vi "ListExamples.vi"(10 "Folder":string) -> (0 "VI Paths":path[](array[path]), 1 "Paths":path[](array[path]), 2 "vis":string[](array[string]), 3 "filenames":string[](array[string]), 5 "folder names":string[](array[string]))   [LabVIEW 2020]
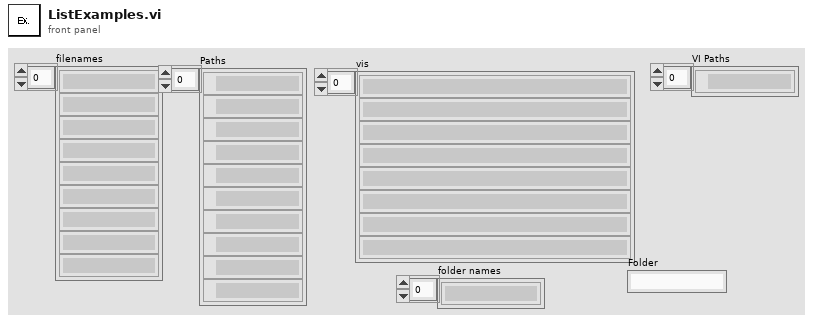
[diagram p1: front panel]
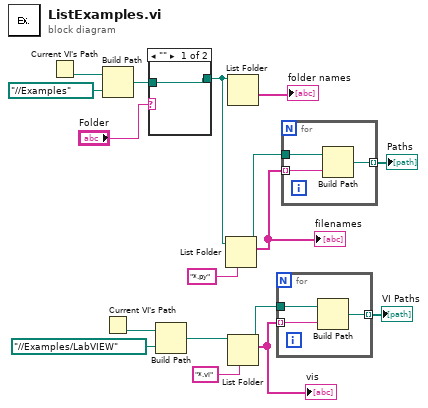
[diagram p0: block diagram]
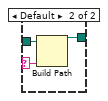
[diagram p2: hidden frame]
diagram:
  n1 = Current VI's Path() -> (path=w5:path)
  n2 = Build Path(base path=w5, name or relative path=path "../../Examples") -> (appended path=w3:path)
  n3 = Current VI's Path() -> (path=w12:path)
  n4 = case shown="\"\"" "Folder" {
    selector: "Folder" -> [_ w19]
    tunnel: w3 -> [w18 w21]
    tunnel: [w18 w20] -> w2
    frame "" {
    }
    frame Default {
      n5 = Build Path(base path=w21, name or relative path=w19) -> (appended path=w20:path)
    }
  }
  n6 = Build Path(base path=w12, name or relative path=path "../../Examples/LabVIEW") -> (appended path=w11:path)
  n7 = List Folder(path=w2, pattern="*.py") -> (path out=w16:path, filenames=w15:string[])  [unwired: 2 in, 2 out]
  "filenames" <- w15
  n8 = List Folder(path=w2) -> (folder names=→"folder names":string[])  [unwired: 3 in, 3 out]
  n9 = List Folder(path=w11, pattern="*.vi") -> (path out=w10:path, filenames=w9:string[])  [unwired: 2 in, 2 out]
  "vis" <- w9
  n10 = for {
    tunnel: w10 -> [w24]
    tunnel: w9 -> [w23] mode=indexing
    tunnel: [w22] -> w8 mode=indexing
    n11 = Build Path(base path=w24, name or relative path=w23) -> (appended path=w22:path)
  }
  "VI Paths" <- w8
  n12 = for {
    tunnel: w16 -> [w27]
    tunnel: w15 -> [w26] mode=indexing
    tunnel: [w25] -> w14 mode=indexing
    n13 = Build Path(base path=w27, name or relative path=w26) -> (appended path=w25:path)
  }
  "Paths" <- w14
